vi "VG_TenmaParam.vi"() -> ()   [LabVIEW 2020]
panel:
  out "Imax":dbl
  out "Imin":dbl
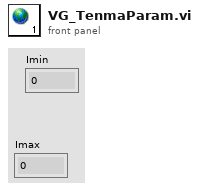
[diagram p1: front panel]
diagram:
